vi "FG Target Sector.vi"(2 "FG Action (Read)":T1, 3 "Target sector in":i16) -> (1 "Target sector out":i16)   [LabVIEW 2009]
uses:
  Actions for FG's.ctl
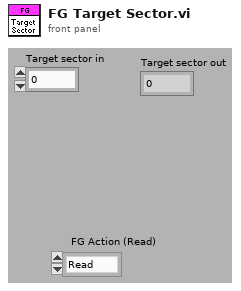
[diagram p1: front panel]
types:
  T1 = typedef "Actions for FG's.ctl" = enum16{"Read", "Write"}
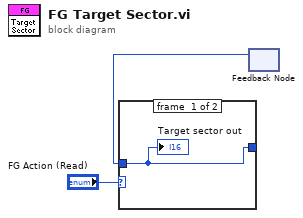
[diagram p0: block diagram]
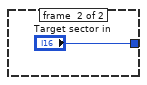
[diagram p2: hidden frame]
diagram:
  n1 = feedback #1() -> (w1:i16)  [unwired: 1 in]
  n2 = case shown="\"Write\"" "FG Action (Read)" {
    tunnel: [w4 "Target sector in"] -> w2
    tunnel: w1 -> [w4 _]
    frame #0 {
      "Target sector out" <- w4
    }
    frame #1 {
    }
  }
